vi "Example Simple DataBinding.vi"() -> ()   [LabVIEW 2014]
doc: "This examples shows off many of the basic usage patterns of the datagrid."
uses:
  System.Windows.Forms
  GridColumn/ColumnDefinition.ctl
  GridColumn/ColumnType.ctl
  DataGridView/DataGridView.lvclass
  DataGrid.lvlib
  Events/CellValueChanged/CellValueChanged.lvclass
  Events/CellClick/CellClick.lvclass
  Events/KeyDown/KeyDown.lvclass
  GridColumn/GridColumn.lvclass
panel:
  out "Events":string
  in  "# of Rows":i32=15
  in  "ColumnSetup":T1[](array[typedef])=[{"name"="Text", "caption"="Text", "datatype"=enum."string", "Params"="", "AutoSizeMode"=2, "FillWeight"=10.0, "MinWidth"=25, "tooltip"="Text The quick brown fox jumps over the lazy dog"}, {"name"="Details", "caption"="Details", "datatype"=enum."string", "Params"="", "AutoSizeMode"=16, "FillWeight"=100.0, "MinWidth"=150, "tooltip"="Details The quick brown fox jumps over the lazy dog"}, {"name"="Time", "caption"="", "datatype"=enum."timestamp", "Params"="", "AutoSizeMode"=1, "FillWeight"=1.0, "MinWidth"=120, "tooltip"="Time The quick brown fox jumps over the lazy dog"}, {"name"="Selection", "caption"="", "datatype"=enum."combo", "Params"="One|Two|Three", "AutoSizeMode"=6, "FillWeight"=1.0, "MinWidth"=80, "tooltip"="Selection The quick brown fox jumps over the lazy dog"}, {"name"="Function", "caption"="", "datatype"=enum."button", "Params"="", "AutoSizeMode"=6, "FillWeight"=1.0, "MinWidth"=50, "tooltip"="Function The quick brown fox jumps over the lazy dog"}, {"name"="Value", "caption"="", "datatype"=enum."numeric", "Params"="", "AutoSizeMode"=6, "FillWeight"=1.0, "MinWidth"=10, "tooltip"="Value The quick brown fox jumps over the lazy dog"}, {"name"="Active", "caption"="", "datatype"=enum."check", "Params"="", "AutoSizeMode"=6, "FillWeight"=1.0, "MinWidth"=10, "tooltip"=""}, {"name"="Status", "caption"="", "datatype"=enum."image", "Params"="", "AutoSizeMode"=6, "FillWeight"=1.0, "MinWidth"=10, "tooltip"=""}, {"name"="Link", "caption"="", "datatype"=enum."link", "Params"="", "AutoSizeMode"=1, "FillWeight"=100.0, "MinWidth"=50, "tooltip"=""}] {"MinWidth" min=2 step=1; "AutoSizeMode" items=["None"=1, "ColumnHeader"=2, "AllCellsExceptHeader"=4, "AllCells"=6, "DisplayedCellsExceptHeader"=8, "DisplayedCells"=10, "Fill"=16]; "FillWeight" min=1 max=100}
  in  "DataGridView":refnum<k24>(container)
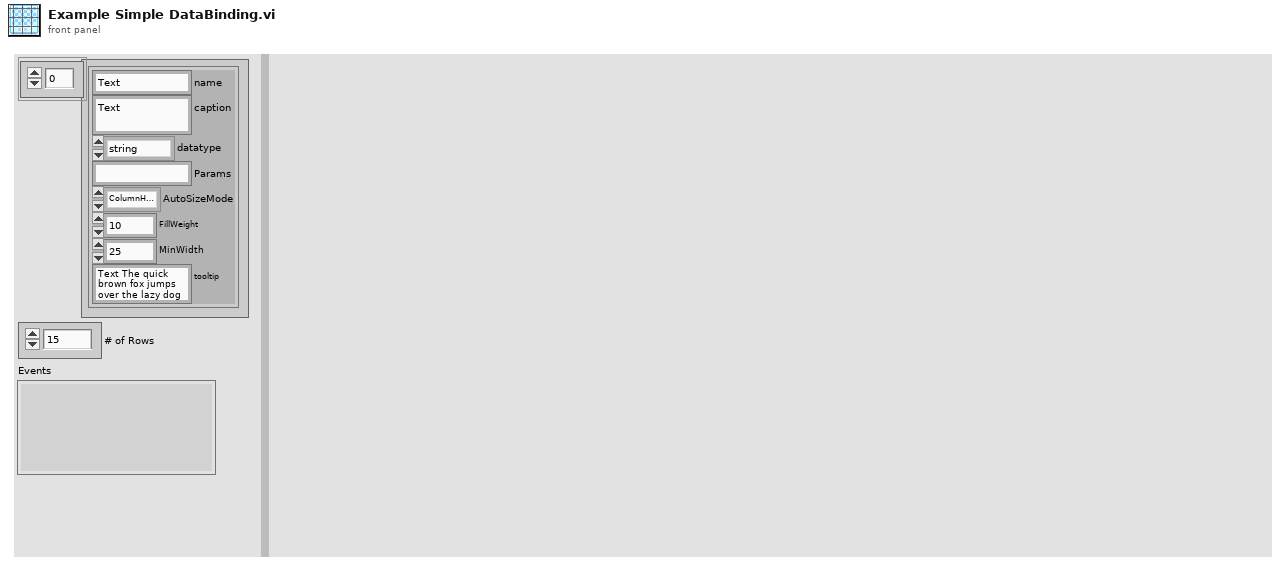
[diagram p1: front panel]
types:
  T1 = typedef "DataGrid.lvlib/GridColumn.lvclass/ColumnDefinition.ctl" = cluster{"name":string, "caption":string, "datatype":T2, "Params":string, "AutoSizeMode":i32, "FillWeight":sgl, "MinWidth":u32, "tooltip":string}
  T2 = typedef "DataGrid.lvlib/GridColumn.lvclass/ColumnType.ctl" = enum16{"string", "image", "check", "numeric", "timestamp", "button", "combo", "link"}
  T3 = cluster{"Alt":bool, "Control":bool, "KeyCode":i32, "KeyData":i32, "KeyValue":i32, "Modifiers":i32, "Shift":bool}
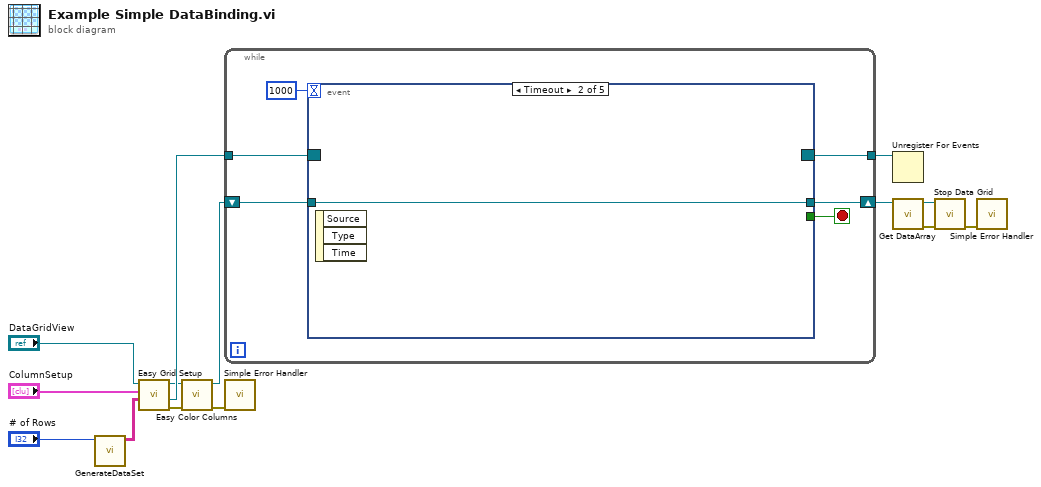
[diagram p0: block diagram]
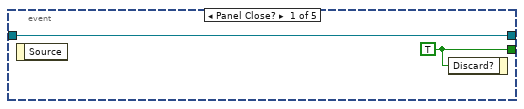
[diagram p2: hidden frame]
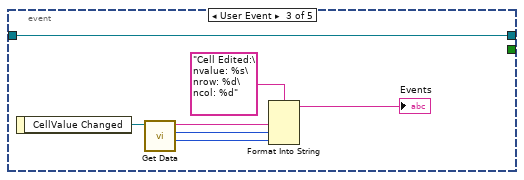
[diagram p3: hidden frame]
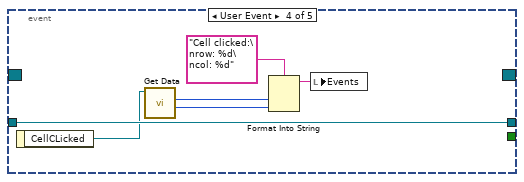
[diagram p4: hidden frame]
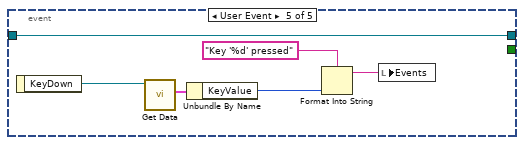
[diagram p5: hidden frame]
diagram:
  n1 = call "GenerateDataSet.vi"("Records"="# of Rows") -> ("DataGrid"=w11:string[][])  [unwired: 10 in]
  n2 = call "Easy Grid Setup.vi"("DataSource Data"=w11, "ColumnSetup"="ColumnSetup", ".net datagridview ref"="DataGridView") -> ("error out"=w9:errorcluster, "registeredEvents"=w10:refnum<event-registration>, "DataGrid out"=w8:refnum<class "DataGridView.lvclass">)  [unwired: 5 in, 1 out]
  n3 = call "Easy Color Columns.vi"("error in (no error)"=w9, "DataGridView in"=w8) -> ("error out"=w7:errorcluster, "DataGridView out"=w6:refnum<class "DataGridView.lvclass">)  [unwired: 8 in]
  n4 = while {
    tunnel: w10 -> [w19]
    shift-right: [w17] -> w3
    shift-left: w6 -> [w18]
    tunnel: [w16] -> w5
    stop <- w20 stop-if-true
    n5 = event shown="[1] Timeout" {
      selector: w19 -> [_ _ _ _ _]
      dyn-events: [_ _ _ _ _] -> w16
      timeout: 1000 -> [_ _ _ _ _]
      tunnel: [w22 _ _ _ _] -> w20
      tunnel: w18 -> [w21 w23 w28 w35 w42]
      tunnel: [w21 w23 w28 w35 w42] -> w17
      event Panel Close? {
        w22 = TRUE ("Discard?")
        n6 = event-data() -> ()  [unwired: 1 in, 1 out]
        n7 = event-data("Discard?"=w22) -> ()  [unwired: 1 in, 1 out]
      }
      event Timeout {
        n8 = event-data() -> ()  [unwired: 1 in, 3 out]
      }
      event User Event {
        n9 = event-data() -> ("CellValue Changed"=w27:refnum<class "Abstract EVENT.lvclass">)  [unwired: 1 in]
        n10 = call "Get Data.vi"("DataGrid.lvlib:Abstract EVENT.lvclass"=w27) -> ("column"=w24:i32, "row"=w25:i32, "cell value"=w26:string)  [unwired: 7 in, 1 out]
        n11 = Format Into String(format string="Cell Edited:\nvalue: %s\nrow: %d\ncol: %d" ("message"), w26, w25, w24) -> (resulting string=→"Events":string)  [unwired: 2 in, 1 out]
      }
      event User Event {
        n12 = event-data() -> ("CellCLicked"=w33:refnum<class "Abstract EVENT.lvclass">)  [unwired: 1 in]
        n13 = call "Get Data.vi"("DataGrid.lvlib:Abstract EVENT.lvclass"=w33) -> ("column"=w31:i32, "row"=w32:i32)  [unwired: 8 in, 1 out]
        n14 = Format Into String(format string="Cell clicked:\nrow: %d\ncol: %d" ("message"), w32, w31) -> (resulting string=w36:string)  [unwired: 2 in, 1 out]
        n15 = local write "Events"(w36) -> ()
      }
      event User Event {
        n16 = event-data() -> ("KeyDown"=w41:refnum<class "Abstract EVENT.lvclass">)  [unwired: 1 in]
        n17 = call "Get Data.vi"("DataGrid.lvlib:Abstract EVENT.lvclass"=w41) -> ("output cluster"=w38:T3)  [unwired: 9 in, 1 out]
        n18 = Unbundle By Name(w38) -> ("KeyValue"=w37:i32)
        n19 = Format Into String(format string="Key '%d' pressed" ("message"), w37) -> (resulting string=w40:string)  [unwired: 2 in, 1 out]
        n20 = local write "Events"(w40) -> ()
      }
    }
  }
  n21 = call <vilib>:"Simple Error Handler.vi"("error in (no error)"=w7) -> ()  [unwired: 4 in, 5 out]
  n22 = Unregister For Events(event registration refnum=w5) -> ()  [unwired: 1 in, 1 out]
  n23 = call "Get DataArray.vi"("DataGridView in"=w3) -> ("error out"=w2:errorcluster, "DataGridView out"=w1:refnum<class "DataGridView.lvclass">)  [unwired: 8 in, 1 out]
  n24 = call "Stop Data Grid.vi"("error in (no error)"=w2, "DataGridView in"=w1) -> ("error out"=w4:errorcluster)  [unwired: 8 in, 1 out]
  n25 = call <vilib>:"Simple Error Handler.vi"("error in (no error)"=w4) -> ()  [unwired: 4 in, 5 out]
